vi "MUSIQC_trap_control_trap2backup.vi"() -> ()   [LabVIEW 2012]
uses:
  Control 1.ctl
  <vilib>/DAQmx/read.llb/DAQmx Read (Counter U32 1Chan 1Samp).vi
  <vilib>/DAQmx/create/channels.llb/DAQmx Create Channel (CO-Pulse Generation-Frequency).vi
  <vilib>/DAQmx/configure/timing.llb/DAQmx Timing (Implicit).vi
  <vilib>/DAQmx/create/channels.llb/DAQmx Create Channel (CI-Count Edges).vi
  <vilib>/DAQmx/configure/timing.llb/DAQmx Timing (Sample Clock).vi
  <vilib>/Analysis/baseanly.llb/Mean (DBL).vi
  <vilib>/DAQmx/miscellaneous.llb/DAQmx Fill In Error Info.vi
  <vilib>/Utility/file.llb/Write To Spreadsheet File (I64).vi
  <resource>/objmgr/daqmx.rc
  <vilib>/Analysis/NI_AALBase.lvlib
panel:
  in  "X window size":dbl=5.0
  out "Sample Rate":dbl
  out "PMT Counts 2":cluster{"mean":dbl, u32, "mean":dbl}(graph)={"mean"=45.0, 28, "mean"=44.815}
  in  "y":bool
  out "x":dbl=70.0
  in  "Samples per averaging\nblock 2":i32=200 min=1 step=1
  in  "UV firing rate":dbl=2.0
  in  "Pockel":bool=TRUE
  in  "Dump Frequency":dbl
  in  "AutoDump":bool
  out "Loading Elapsed Time":dbl
  out "Loading Start Time":timestamp=timestamp(3525114376.279 s since 1904-01-01)
  in  "UV":bool
  in  "1762":bool
  in  "455 LED":bool
  in  "399 Yb Ionizer":bool
  in  "Oven":bool
  in  "Orange":bool=TRUE
  in  "Sample Time":dbl=0.02 format="%0.2f"
  in  "snap":bool
  in  "Threshold":u32
  in  "Auto Load":bool
  in  "RF":bool
  in  "Blue":bool=TRUE
  in  "Red":bool=TRUE
  out "Mean":T1=45.0 format="%0.2d"
  in  "Samples per averaging\nblock":i32=20 min=1 step=1
  in  "stop":bool
  out "PMT Counts":cluster{"mean":dbl, u32, "mean":dbl}(graph)={"mean"=45.0, 28, "mean"=44.815}
  out "Counts total":dbl=75014.0
  # "Trap 2"
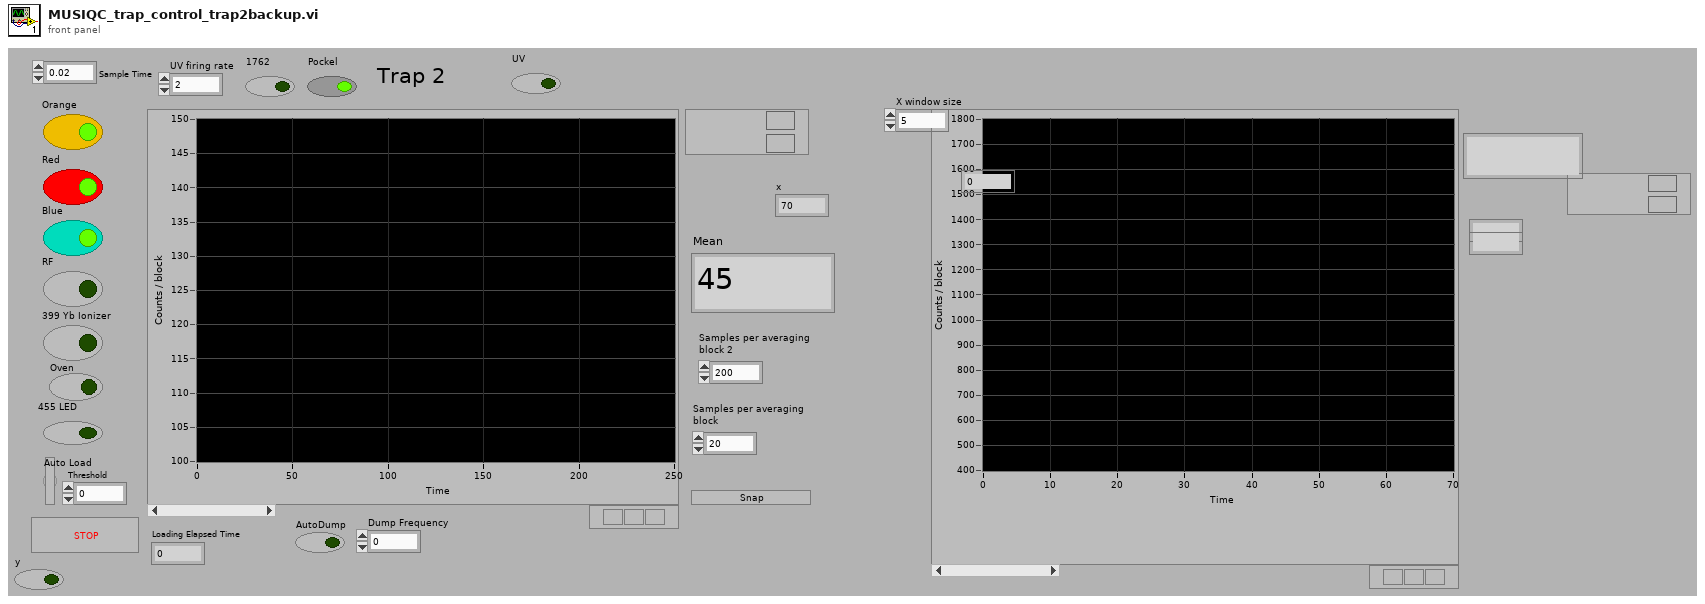
[diagram p1: front panel]
types:
  T1 = typedef "Control 1.ctl" = dbl
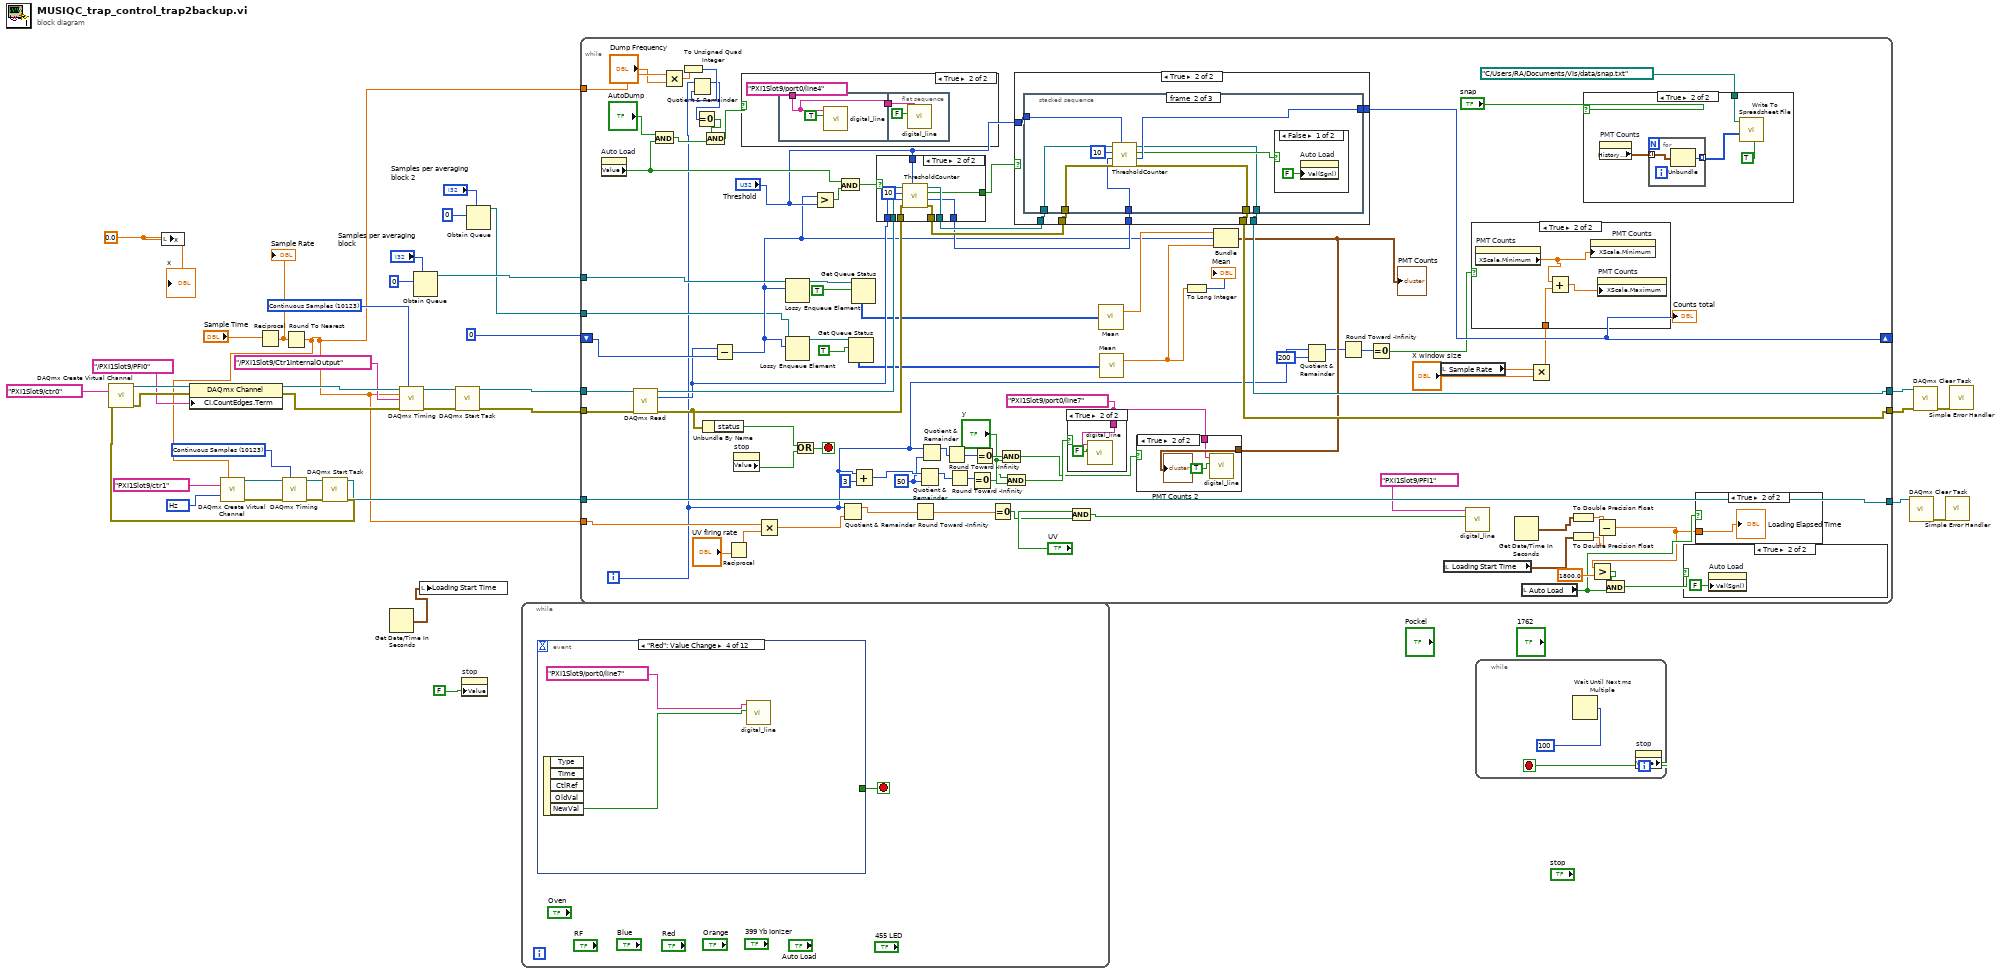
[diagram p0: block diagram]
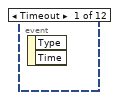
[diagram p2: hidden frame]
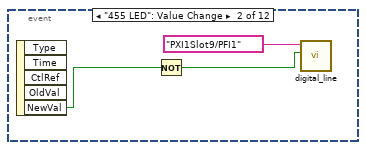
[diagram p3: hidden frame]
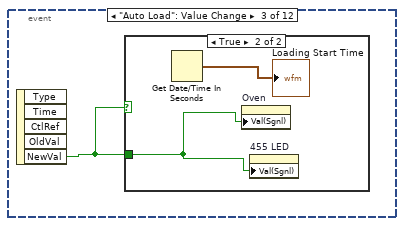
[diagram p4: hidden frame]
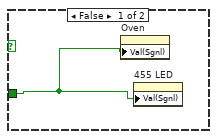
[diagram p5: hidden frame]
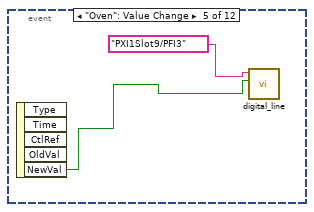
[diagram p6: hidden frame]
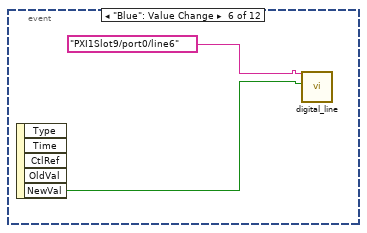
[diagram p7: hidden frame]
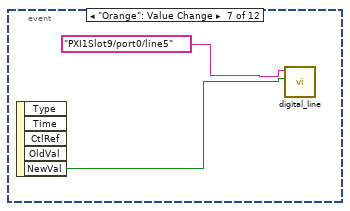
[diagram p8: hidden frame]
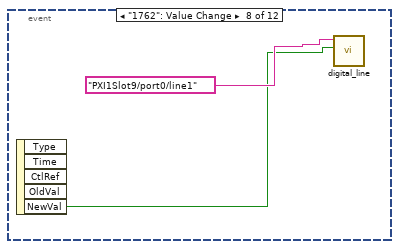
[diagram p9: hidden frame]
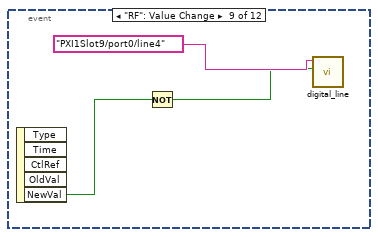
[diagram p10: hidden frame]
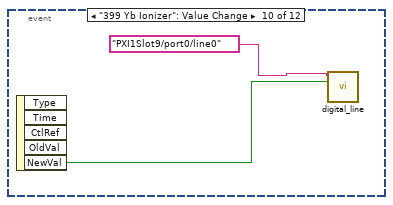
[diagram p11: hidden frame]
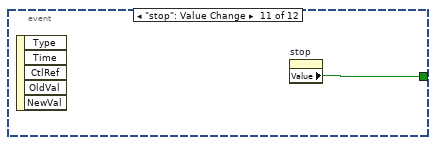
[diagram p12: hidden frame]
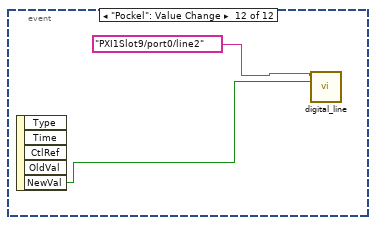
[diagram p13: hidden frame]
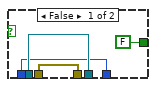
[diagram p17: hidden frame]
diagram:
  w1 = 0.0 ("x")
  w9 = 10123 items=["Finite Samples"=10178, "Continuous Samples"=10123, "Hardware Timed Single Point"=12522] ("sample mode")
  w16 = 10373 items=["Hz"=10373] ("units")
  w22 = 10123 items=["Finite Samples"=10178, "Continuous Samples"=10123, "Hardware Timed Single Point"=12522] ("sample mode")
  n1 = local write "x"(w1) -> ()
  n2 = Reciprocal(x="Sample Time") -> (1/x=w6:dbl)
  "Sample Rate" <- w6
  n3 = Round To Nearest(number=w6) -> (nearest integer value=w5:dbl)
  n4 = call-poly <vilib>:"DAQmx Create Virtual Channel.vi"("frequency"=w5, "counter"=tag "PXI1Slot9/ctr1", "units"=w16) -> ("task out"=w13:refnum<k21>, "error out"=w12:errorcluster)  [unwired: 11 in]
  n5 = call-poly <vilib>:"DAQmx Timing.vi"("task/channels in"=w13, "sample mode"=w9, "error in"=w12) -> ("task out"=w11:refnum<k21>, "error out"=w10:errorcluster)  [unwired: 11 in]
  n6 = call <vilib>:"DAQmx Start Task.vi"("task/channels in"=w11, "error in"=w10) -> ("task out"=w19:refnum<k21>, "error out"=w20:errorcluster)  [unwired: 12 in]
  n7 = call-poly <vilib>:"DAQmx Create Virtual Channel.vi"("counter"=tag "PXI1Slot9/ctr0", "error in"=w20) -> ("task out"=w30:refnum<k21>, "error out"=w29:errorcluster)  [unwired: 12 in]
  n8 = property class="DAQmx Channel"(reference=w30, error in=w29, "CI.CountEdges.Term"=tag "/PXI1Slot9/PFI0") -> (reference out=w32:refnum<k21>, error out=w31:errorcluster)
  n9 = Get Date/Time In Seconds() -> (seconds since 1Jan1904=w8:timestamp)
  n10 = call-poly <vilib>:"DAQmx Timing.vi"("task/channels in"=w32, "sample mode"=w22, "rate"=w5, "source"=tag "/PXI1Slot9/Ctr1InternalOutput", "error in"=w31) -> ("task out"=w38:refnum<k21>, "error out"=w37:errorcluster)  [unwired: 9 in]
  n11 = Obtain Queue(max queue size (-1, unlimited)="Samples per averaging\nblock", element data type=u32 0) -> (queue out=w25:refnum<queue>)  [unwired: 3 in, 2 out]
  n12 = local write "Loading Start Time"(w8) -> ()
  n13 = call <vilib>:"DAQmx Start Task.vi"("task/channels in"=w38, "error in"=w37) -> ("task out"=w33:refnum<k21>, "error out"=w15:errorcluster)  [unwired: 12 in]
  n14 = property on="stop" class="Bool (strict)"("Value"=FALSE ("stop")) -> ()  [unwired: 2 in, 2 out]
  n15 = Obtain Queue(max queue size (-1, unlimited)="Samples per averaging\nblock 2", element data type=u32 0) -> (queue out=w2:refnum<queue>)  [unwired: 3 in, 2 out]
  n16 = while {
    stop <- w40 stop-if-true
    n17 = event shown="[3] \"Red\": Value Change" {
      selector: _ -> [_ _ _ _ _ _ _ _ _ _ _ _]
      dyn-events: _ -> [_ _ _ _ _ _ _ _ _ _ _ _]
      timeout: _ -> [_ _ _ _ _ _ _ _ _ _ _ _]
      tunnel: [_ _ _ _ _ _ _ _ _ _ w63 _] -> w40
      event Timeout {
        n18 = event-data() -> ()  [unwired: 1 in, 2 out]
      }
      event "455 LED": Value Change {
        n19 = event-data() -> ("NewVal"=w43:bool)  [unwired: 1 in, 4 out]
        n20 = Not(x=w43) -> (.not. x?=w41:bool)
        n21 = call "digital_line.vi"("Boolean"=w41, "lines"=tag "PXI1Slot9/PFI1") -> ()  [unwired: 5 in, 1 out]
      }
      event "Auto Load": Value Change {
        n22 = event-data() -> ("NewVal"=w44:bool)  [unwired: 1 in, 4 out]
        n23 = case shown="True" w44 {
          tunnel: w44 -> [w45 w46]
          frame False {
            n24 = property on="Oven" class="Bool (strict)"("Val(Sgnl)"=w45) -> ()  [unwired: 2 in, 2 out]
            n25 = property on="455 LED" class="Bool (strict)"("Val(Sgnl)"=w45) -> ()  [unwired: 2 in, 2 out]
          }
          frame True {
            n26 = Get Date/Time In Seconds() -> (seconds since 1Jan1904=→"Loading Start Time":timestamp)
            n27 = property on="Oven" class="Bool (strict)"("Val(Sgnl)"=w46) -> ()  [unwired: 2 in, 2 out]
            n28 = property on="455 LED" class="Bool (strict)"("Val(Sgnl)"=w46) -> ()  [unwired: 2 in, 2 out]
          }
        }
      }
      event "Red": Value Change {
        n29 = event-data() -> ("NewVal"=w48:bool)  [unwired: 1 in, 4 out]
        n30 = call "digital_line.vi"("Boolean"=w48, "lines"=tag "PXI1Slot9/port0/line7") -> ()  [unwired: 5 in, 1 out]
      }
      event "Oven": Value Change {
        n31 = event-data() -> ("NewVal"=w50:bool)  [unwired: 1 in, 4 out]
        n32 = call "digital_line.vi"("Boolean"=w50, "lines"=tag "PXI1Slot9/PFI3") -> ()  [unwired: 5 in, 1 out]
      }
      event "Blue": Value Change {
        n33 = event-data() -> ("NewVal"=w52:bool)  [unwired: 1 in, 4 out]
        n34 = call "digital_line.vi"("Boolean"=w52, "lines"=tag "PXI1Slot9/port0/line6") -> ()  [unwired: 5 in, 1 out]
      }
      event "Orange": Value Change {
        n35 = event-data() -> ("NewVal"=w54:bool)  [unwired: 1 in, 4 out]
        n36 = call "digital_line.vi"("Boolean"=w54, "lines"=tag "PXI1Slot9/port0/line5") -> ()  [unwired: 5 in, 1 out]
      }
      event "1762": Value Change {
        n37 = event-data() -> ("NewVal"=w56:bool)  [unwired: 1 in, 4 out]
        n38 = call "digital_line.vi"("Boolean"=w56, "lines"=tag "PXI1Slot9/port0/line1") -> ()  [unwired: 5 in, 1 out]
      }
      event "RF": Value Change {
        n39 = event-data() -> ("NewVal"=w60:bool)  [unwired: 1 in, 4 out]
        n40 = Not(x=w60) -> (.not. x?=w58:bool)
        n41 = call "digital_line.vi"("Boolean"=w58, "lines"=tag "PXI1Slot9/port0/line4") -> ()  [unwired: 5 in, 1 out]
      }
      event "399 Yb Ionizer": Value Change {
        n42 = event-data() -> ("NewVal"=w61:bool)  [unwired: 1 in, 4 out]
        n43 = call "digital_line.vi"("Boolean"=w61, "lines"=tag "PXI1Slot9/port0/line0") -> ()  [unwired: 5 in, 1 out]
      }
      event "stop": Value Change {
        n44 = event-data() -> ()  [unwired: 1 in, 5 out]
        n45 = property on="stop" class="Bool (strict)"() -> ("Value"=w63:bool)  [unwired: 2 in, 2 out]
      }
      event "Pockel": Value Change {
        n46 = event-data() -> ("NewVal"=w64:bool)  [unwired: 1 in, 4 out]
        n47 = call "digital_line.vi"("Boolean"=w64, "lines"=tag "PXI1Slot9/port0/line2") -> ()  [unwired: 5 in, 1 out]
      }
    }
  }
  n48 = while {
    shift-right: [w111] -> _
    shift-left: u32 0 -> [w140]
    tunnel: [w112] -> w35
    tunnel: [w113] -> w34
    tunnel: w33 -> [w148]
    tunnel: w25 -> [w147]
    tunnel: w19 -> [w139]
    tunnel: [w139] -> w17
    tunnel: w15 -> [w138]
    tunnel: w5 -> [w101]
    tunnel: w5 -> [w122]
    tunnel: w2 -> [w93]
    i -> [w73]
    stop <- w150 stop-if-true
    w76 = tag "PXI1Slot9/port0/line7" ("lines")
    w85 = 50 ("y")
    n49 = property on="Auto Load" class="Bool (strict)"() -> ("Value"=w117:bool)  [unwired: 2 in, 2 out]
    n50 = call-poly <vilib>:"DAQmx Read.vi"("task/channels in"=w148, "error in"=w138) -> ("task out"=w109:refnum<k21>, "data"=w105:u32, "error out"=w108:errorcluster)  [unwired: 11 in]
    n51 = And(x="AutoDump", y=w117) -> (x .and. y?=w115:bool)
    n52 = Multiply(x=w122, y="Dump Frequency") -> (x*y=w120:dbl)
    n53 = To Unsigned Quad Integer(1:w120) -> (0:w119:u64)
    n54 = Quotient & Remainder(x=w73, y=w119) -> (x-y*floor(x/y)=w118:u64)  [unwired: 1 out]
    n55 = Equal To 0?(x=w118) -> (x = 0?=w116:bool)
    n56 = Unbundle By Name(w108) -> ("status"=w149:bool)
    n57 = And(x=w116, y=w115) -> (x .and. y?=w114:bool)
    n58 = Subtract(x=w105, y=w140) -> (x-y=w94:u32)
    n59 = Reciprocal(x="UV firing rate") -> (1/x=w98:dbl)
    n60 = property on="stop" class="Bool (strict)"() -> ("Value"=w144:bool)  [unwired: 2 in, 2 out]
    n61 = case shown="True" w114 {
      frame False {
      }
      frame True {
        n62 = flat-sequence {
          tunnel: tag "PXI1Slot9/port0/line4" ("lines") -> [w175]
          tunnel: [w175] -> w172
          tunnel: w172 -> [w177]
          frame #0 {
            n63 = call "digital_line.vi"("Boolean"=TRUE, "lines"=w175) -> ()  [unwired: 5 in, 1 out]
          }
          frame #1 {
            n64 = call "digital_line.vi"("Boolean"=FALSE, "lines"=w177) -> ()  [unwired: 5 in, 1 out]
          }
        }
      }
    }
    n65 = Multiply(x=w101, y=w98) -> (x*y=w97:dbl)
    n66 = Lossy Enqueue Element(queue=w147, element=w94) -> (queue out=w146:refnum<queue>)  [unwired: 1 in, 3 out]
    n67 = Lossy Enqueue Element(queue=w93, element=w94) -> (queue out=w92:refnum<queue>)  [unwired: 1 in, 3 out]
    n68 = Or(x=w149, y=w144) -> (x .or. y?=w150:bool)
    n69 = Greater?(x=w94, y="Threshold") -> (0:w143:bool)
    n70 = And(x=w117, y=w143) -> (x .and. y?=w110:bool)
    n71 = Quotient & Remainder(x=w73, y=w97) -> (x-y*floor(x/y)=w137:dbl)  [unwired: 1 out]
    n72 = Get Queue Status(queue=w92, return elements? (F)=TRUE) -> (elements=w90:u32[])  [unwired: 1 in, 7 out]
    n73 = Get Queue Status(queue=w146, return elements? (F)=TRUE) -> (elements=w91:u32[])  [unwired: 1 in, 7 out]
    n74 = Add(x=w73, y=3) -> (x+y=w86:i32)
    n75 = case shown="True" w110 {
      tunnel: w109 -> [w160 w171]
      tunnel: w108 -> [w161 w170]
      tunnel: [w161 w169] -> w107
      tunnel: [w160 w168] -> w106
      tunnel: w105 -> [w159 w166]
      tunnel: [w159 w165] -> w104
      tunnel: [FALSE ("Over Threshold") w164] -> w103
      tunnel: "Threshold" -> [_ w163]
      frame False {
      }
      frame True {
        n76 = call "ThresholdCounter.vi"("Threshold"=w163, "error in"=w170, "Previous Counter"=w166, "number of samples per channel"=10, "task/channels in"=w171) -> ("error out"=w169:errorcluster, "Final Counter"=w165:u32, "Over Threshold"=w164:bool, "task out"=w168:refnum<k21>)  [unwired: 3 in]
      }
    }
    n77 = Round Toward -Infinity(1:w137) -> (0:w100:dbl)
    n78 = Quotient & Remainder(x=w86, y=w85) -> (x-y*floor(x/y)=w84:i32)  [unwired: 1 out]
    n79 = Quotient & Remainder(x=w73, y=w85) -> (x-y*floor(x/y)=w83:i32)  [unwired: 1 out]
    n80 = Round Toward -Infinity(1:w83) -> (0:w82:i32)
    n81 = Round Toward -Infinity(1:w84) -> (0:w81:i32)
    n82 = Equal To 0?(x=w81) -> (x = 0?=w78:bool)
    n83 = Equal To 0?(x=w82) -> (x = 0?=w80:bool)
    n84 = Equal To 0?(x=w100) -> (x = 0?=w135:bool)
    n85 = And(x=w80, y="y") -> (x .and. y?=w74:bool)
    n86 = And(x=w78, y="y") -> (x .and. y?=w75:bool)
    n87 = case shown="True" w103 {
      tunnel: w106 -> [w187 w195]
      tunnel: w107 -> [w188 w194]
      tunnel: [w187 w193] -> w113
      tunnel: [w188 w192] -> w112
      tunnel: "Threshold" -> [_ w191]
      tunnel: w104 -> [w186 w190]
      tunnel: [w186 w189] -> w111
      frame False {
      }
      frame True {
        n88 = stacked-sequence {
          tunnel: w195 -> [_ w206 _]
          tunnel: w194 -> [_ w205 _]
          tunnel: [_ w199 _] -> w193
          tunnel: [_ w200 _] -> w192
          tunnel: w191 -> [_ w198 _]
          tunnel: w190 -> [_ w203 _]
          tunnel: [_ w202 _] -> w189
          frame #0 {
            n89 = call "digital_line.vi"("Boolean"=FALSE, "lines"=tag "PXI1Slot9/port0/line7") -> ()  [unwired: 5 in, 1 out]
          }
          frame #1 {
            n90 = call "ThresholdCounter.vi"("Threshold"=w198, "error in"=w205, "Previous Counter"=w203, "number of samples per channel"=10, "task/channels in"=w206) -> ("error out"=w200:errorcluster, "Final Counter"=w202:u32, "Over Threshold"=w201:bool, "task out"=w199:refnum<k21>)  [unwired: 3 in]
            n91 = case shown="False" w201 {
              frame False {
                n92 = property on="Auto Load" class="Bool (strict)"("Val(Sgnl)"=FALSE ("Auto Load")) -> ()  [unwired: 2 in, 2 out]
              }
              frame True {
              }
            }
          }
          frame #2 {
            n93 = call "digital_line.vi"("Boolean"=TRUE, "lines"=tag "PXI1Slot9/port0/line7") -> ()  [unwired: 5 in, 1 out]
          }
        }
      }
    }
    "Counts total" <- w111
    n94 = case shown="True" w75 {
      tunnel: w76 -> [_ w158]
      frame False {
      }
      frame True {
        n95 = call "digital_line.vi"("Boolean"=FALSE, "lines"=w158) -> ()  [unwired: 5 in, 1 out]
      }
    }
    n96 = And(x="UV", y=w135) -> (x .and. y?=w133:bool)
    n97 = call-poly <vilib>:"Mean.vi"("X"=w91) -> ("mean"=w145:dbl)  [unwired: 1 out]
    n98 = call-poly <vilib>:"Mean.vi"("X"=w90) -> ("mean"=w89:dbl)  [unwired: 1 out]
    n99 = To Long Integer(number=w89) -> (32bit integer=→"Mean":i32)
    n100 = Bundle("mean"=w145, w94, "mean"=w89) -> (w77:cluster{"mean":dbl, u32, "mean":dbl})  [unwired: 1 in]
    "PMT Counts" <- w77
    n101 = case shown="True" w74 {
      tunnel: w77 -> [_ w155]
      tunnel: w76 -> [_ w154]
      frame False {
      }
      frame True {
        n102 = call "digital_line.vi"("Boolean"=TRUE, "lines"=w154) -> ()  [unwired: 5 in, 1 out]
        "PMT Counts 2" <- w155
      }
    }
    n103 = Quotient & Remainder(x=w73, y=200) -> (x-y*floor(x/y)=w71:i32)  [unwired: 1 out]
    n104 = Round Toward -Infinity(1:w71) -> (0:w70:i32)
    n105 = Equal To 0?(x=w70) -> (x = 0?=w69:bool)
    n106 = local read "Sample Rate"() -> (w68:dbl)
    n107 = local read "Loading Start Time"() -> (w128:timestamp)
    n108 = call "digital_line.vi"("Boolean"=w133, "lines"=tag "PXI1Slot9/PFI1") -> ()  [unwired: 5 in, 1 out]
    n109 = Get Date/Time In Seconds() -> (seconds since 1Jan1904=w131:timestamp)
    n110 = local read "Auto Load"() -> (w125:bool)
    n111 = Multiply(x=w68, y="X window size") -> (x*y=w66:dbl)
    n112 = case shown="True" w69 {
      tunnel: w66 -> [_ w151]
      frame False {
      }
      frame True {
        n113 = property on="PMT Counts" class="WFChart (strict)"() -> ("XScale.Minimum"=w153:dbl)  [unwired: 2 in, 2 out]
        n114 = Add(x=w153, y=w151) -> (x+y=w152:dbl)
        n115 = property on="PMT Counts" class="WFChart (strict)"("XScale.Minimum"=w153) -> ()  [unwired: 2 in, 2 out]
        n116 = property on="PMT Counts" class="WFChart (strict)"("XScale.Maximum"=w152) -> ()  [unwired: 2 in, 2 out]
      }
    }
    n117 = To Double Precision Float(number=w131) -> (double precision float=w129:dbl)
    n118 = To Double Precision Float(number=w128) -> (double precision float=w130:dbl)
    n119 = case shown="True" "snap" {
      tunnel: path "C:/Users/RA/Documents/VIs/data/snap.txt" ("file path (dialog if empty)") -> [_ w182]
      frame False {
      }
      frame True {
        n120 = property on="PMT Counts" class="WFChart (strict)"() -> ("History Data"=w181:cluster{"mean":dbl, u32, "mean":dbl}[])  [unwired: 2 in, 2 out]
        n121 = for {
          tunnel: w181 -> [w185] mode=indexing
          tunnel: [w184] -> w180 mode=indexing
          n122 = Unbundle(w185) -> (w184:u32)  [unwired: 2 out]
        }
        n123 = call-poly <vilib>:"Write To Spreadsheet File.vi"("transpose? (no:F)"=TRUE, "1D data"=w180, "file path (dialog if empty)"=w182) -> ()  [unwired: 5 in, 1 out]
      }
    }
    n124 = Subtract(x=w129, y=w130) -> (x-y=w124:dbl)
    n125 = Greater?(x=w124, y=1800.0) -> (0:w127:bool)
    n126 = And(x=w127, y=w125) -> (x .and. y?=w126:bool)
    n127 = case shown="True" w126 {
      frame False {
      }
      frame True {
        n128 = property on="Auto Load" class="Bool (strict)"("Val(Sgnl)"=FALSE ("Value (Signaling)")) -> ()  [unwired: 2 in, 2 out]
      }
    }
    n129 = case shown="True" w125 {
      tunnel: w124 -> [_ w178]
      frame False {
      }
      frame True {
        "Loading Elapsed Time" <- w178
      }
    }
  }
  n130 = while {
    stop <- w210 stop-if-true
    n131 = Wait Until Next ms Multiple(millisecond multiple=u32 100) -> ()  [unwired: 1 out]
    n132 = property on="stop" class="Bool (strict)"() -> ("Value"=w210:bool)  [unwired: 2 in, 2 out]
  }
  n133 = call <vilib>:"DAQmx Clear Task.vi"("task in"=w17) -> ("error out"=w18:errorcluster)  [unwired: 14 in]
  n134 = call <vilib>:"DAQmx Clear Task.vi"("task in"=w34, "error in"=w35) -> ("error out"=w23:errorcluster)  [unwired: 13 in]
  n135 = call <vilib>:"Simple Error Handler.vi"("error in (no error)"=w18) -> ()  [unwired: 4 in, 5 out]
  n136 = call <vilib>:"Simple Error Handler.vi"("error in (no error)"=w23) -> ()  [unwired: 4 in, 5 out]
  "x" <- w1
